vi "HFRR ADV v05 new software.vi"() -> ()   [LabVIEW 2025] (continued)
        n2735 = case shown="True" "OK Button 17" {
          frame False {
          }
          frame True {
            (unwired) 0  # existing file
            w3786 = "Choose a datalog file to open"  # prompt
            n2736 = local write "OK Button 17"(FALSE ("OK Button 17")) -> ()
            n2737 = local read "String"() -> (w3781:string)
            n2738 = String To Path(string=w3781) -> (path=w3782:path)
            n2739 = File Dialog(6:"*.duf" ("pattern"), 7:w3786, 11:w3782) -> (0:w3773:errorcluster, 3:w3792:path)  [unwired: 4 in, 2 out]
            n2740 = Unbundle(w3773) -> ()  [unwired: 3 out]
            n2741 = Open/Create/Replace File "Open File"(file path (use dialog)=w3792) -> (refnum out=w3784:refnum<file>)  [unwired: 5 in, 2 out]
            n2742 = Strip Path(path=w3792) -> (name=w3790:string)  [unwired: 1 out]
            n2743 = Path To String(path=w3792) -> (string=w3775:string)
            n2744 = while {
              tunnel: w3784 -> [w3796]
              i -> [w3793]
              stop <- w3794 continue-if-true
              (unwired) TRUE ("line mode (F)")
              n2745 = Read from Text File "Read File"(file (use dialog)=w3796) -> (text=w3795:string)  [unwired: 3 in, 3 out]
              n2746 = local write "Numeric 16"(w3793) -> ()
              n2747 = String Length(string=w3795) -> (length=w3798:i32)
              n2748 = Greater?(x=w3798, y=1) -> (0:w3794:bool)
            }
            n2749 = local write "String 29"(w3775) -> ()
            n2750 = Search and Replace String(input string=w3775, search string=".duf", replace string=".dgf" ("replace string (\"\")")) -> (result string=→"String Indicator 4":string)  [unwired: 5 in, 3 out]
            n2751 = Match Pattern(string=w3790, regular expression=".dwm") -> (before substring=w3774:string)  [unwired: 1 in, 3 out]
            "String Indicator" <- w3774
            n2752 = Match Pattern(string=w3775, regular expression=".dwm" ("substring (\"\")")) -> (before substring=w3776:string)  [unwired: 1 in, 3 out]
            "String Indicator 3" <- w3776
            n2753 = local write "TITTLE 2"(w3774) -> ()
            n2754 = String To Path(string=w3776) -> (path=w3783:path)
            "path" <- w3783
            n2755 = call <vilib>:"Read Characters From File.vi"("file path (dialog if empty)"=w3783, "start of read offset (chars.:0)"=60 ("start of read offset (chars.: 0)")) -> ("character string"=→"String Indicator 2":string)  [unwired: 4 in, 3 out]
          }
        }
        n2756 = call <vilib>:"Query Available Printers.vi"() -> ("system configured printers"=w3475:string[])  [unwired: 9 in, 2 out]
        "System Configured Printers 2" <- w3475
        n2757 = local read "OK Button 16"() -> (w3472:bool)
        n2758 = case shown="True" "OK Button 16" {
          frame False {
          }
          frame True {
            n2759 = stacked-sequence {
              frame #0 {
                n2760 = local read "Numeric 16"() -> (w3800:i32)
                n2761 = local write "Numeric 10"(w3800) -> ()
              }
              frame #1 {
                n2762 = local read "S.NO"() -> (→"s.NO":string)
                n2763 = local read "String 29"() -> (w3804:string)
                n2764 = String To Path(string=w3804) -> (path=w3803:path)
                n2765 = Open/Create/Replace File "Open File"(file path (use dialog)=w3803) -> (refnum out=w3805:refnum<file>)  [unwired: 5 in, 2 out]
                n2766 = for {
                  N: 16 -> [_]
                  tunnel: w3805 -> [w3812]
                  i -> [w3808]
                  (unwired) TRUE ("line mode (F)")
                  n2767 = Read from Text File "Read File"(file (use dialog)=w3812) -> (text=w3806:string)  [unwired: 3 in, 3 out]
                  n2768 = Match Pattern(string=w3806, regular expression="(") -> (after substring=w3811:string)  [unwired: 1 in, 3 out]
                  n2769 = Match Pattern(string=w3811, regular expression=")") -> (before substring=w3807:string)  [unwired: 1 in, 3 out]
                  n2770 = case shown="1" w3808 {
                    tunnel: w3807 -> [w3813 w3814 _ _ w3815 w3816 w3817 w3819 w3821 w3823 w3825 w3827 w3829 w3831 _]
                    tunnel: w3806 -> [_ _ _ _ _ _ _ _ _ _ _ _ _ _ _]
                    frame 0 {
                      "TITTLE" <- w3813
                    }
                    frame 1 {
                      "Sample ID" <- w3814
                    }
                    frame 2 {
                    }
                    frame 3 {
                    }
                    frame 4 {
                      "Test Date" <- w3815
                    }
                    frame 5 {
                      "Tested by" <- w3816
                    }
                    frame 6 {
                      n2771 = Fract/Exp String To Number(string=w3817) -> (number=→"Humidity before test 2":dbl)  [unwired: 3 in, 1 out]
                    }
                    frame 7 {
                      n2772 = Fract/Exp String To Number(string=w3819) -> (number=→"Temperature before test 2":dbl)  [unwired: 3 in, 1 out]
                    }
                    frame 8 {
                      n2773 = Fract/Exp String To Number(string=w3821) -> (number=→"Humidity after test 2":dbl)  [unwired: 3 in, 1 out]
                    }
                    frame 9 {
                      n2774 = Fract/Exp String To Number(string=w3823) -> (number=→"Temperature after test 2":dbl)  [unwired: 3 in, 1 out]
                    }
                    frame 10 {
                      n2775 = Fract/Exp String To Number(string=w3825) -> (number=→"MWSD 2":dbl)  [unwired: 3 in, 1 out]
                    }
                    frame 11 {
                      n2776 = Fract/Exp String To Number(string=w3827) -> (number=→"AVP 2":dbl)  [unwired: 3 in, 1 out]
                    }
                    frame 12 {
                      n2777 = Fract/Exp String To Number(string=w3829) -> (number=→"HCF 2":dbl)  [unwired: 3 in, 1 out]
                    }
                    frame 13 {
                      n2778 = Fract/Exp String To Number(string=w3831) -> (number=→"WS1.4 2":dbl)  [unwired: 3 in, 1 out]
                    }
                    frame 14, Default {
                    }
                  }
                }
              }
              frame #2 {
              }
            }
            n2779 = local write "OK Button 16"(FALSE ("OK Button 13")) -> ()
          }
        }
        n2780 = Index Array(array=w3475, index="Select Printer 3") -> (element=w3477:string)
        "Selected Printer" <- w3477
        n2781 = case shown="True" w3472 {
          frame False {
          }
          frame True {
            n2782 = flat-sequence {
              frame #0 {
              }
              frame #1 {
                n2783 = Wait (ms)(milliseconds to wait=u32 100) -> ()  [unwired: 1 out]
              }
              frame #2 {
                n2784 = local write "OK Button 16"(FALSE ("Print 3")) -> ()
              }
            }
          }
        }
        n2785 = case shown="True" "Print" {
          tunnel: w3477 -> [_ w3769]
          frame False {
          }
          frame True {
            (unwired) i16 6 ("width (-)")
            (unwired) "TESTED BY : "
            (unwired) "TESTED DATE :"
            (unwired) "SAMPLE ID : "
            (unwired) "SAMPLE DESIGN : "
            w3727 = "\r"
            w3744 = "\r"
            # "add image"
            n2786 = local read "Sample ID"() -> (w3717:string)
            n2787 = local read "Tested by"() -> (w3720:string)
            n2788 = local read "String 34"() -> (w3707:string)
            n2789 = local read "String 45"() -> (w3687:string)
            n2790 = local read "String 35"() -> (w3702:string)
            n2791 = local read "String 37"() -> (w3700:string)
            n2792 = local read "String 32"() -> (w3722:string)
            n2793 = local read "String 36"() -> (w3697:string)
            n2794 = local read "String 31"() -> (w3721:string)
            n2795 = local read "Test Date"() -> (w3718:string)
            n2796 = local read "String 33"() -> (w3723:string)
            n2797 = local read "String 38"() -> (w3693:string)
            n2798 = local read "String 39"() -> (w3690:string)
            n2799 = local write "Print"(FALSE ("Print FF")) -> ()
            n2800 = local read "S 39"() -> (w3705:string)
            n2801 = local read "S 38"() -> (w3712:string)
            n2802 = local read "Temperature before test 2"() -> (w3743:dbl)
            n2803 = local read "Temperature after test 2"() -> (w3733:dbl)
            n2804 = local read "Humidity before test 2"() -> (w3758:dbl)
            n2805 = local read "Humidity after test 2"() -> (w3742:dbl)
            n2806 = local read "MWSD 2"() -> (w3747:dbl)
            n2807 = local read "WS1.4 2"() -> (w3725:dbl)
            n2808 = Concatenate Strings("2)" ("string"), w3707) -> (w3708:string)
            n2809 = Concatenate Strings("3)" ("string"), w3705) -> (w3706:string)
            n2810 = Concatenate Strings("1)" ("string"), w3712) -> (w3711:string)
            n2811 = Concatenate Strings("4)" ("string"), w3702) -> (w3703:string)
            n2812 = Concatenate Strings("5)" ("string"), w3700) -> (w3699:string)
            n2813 = Concatenate Strings("6)" ("string"), w3697) -> (w3696:string)
            n2814 = Concatenate Strings("7)" ("string"), w3693) -> (w3694:string)
            n2815 = Concatenate Strings("8)" ("string"), w3690) -> (w3691:string)
            n2816 = local read "HCF 2"() -> (w3729:dbl)
            n2817 = local read "AVP 2"() -> (w3746:dbl)
            n2818 = local read "s.NO"() -> (w3688:string)
            n2819 = call <vilib>:"New Report.vi"("report type"=enum16{"Standard Report", "HTML"}."Standard Report") -> ("report out"=w3767:refnum<class "NI_report.lvclass">, "error out"=w3766:errorcluster)  [unwired: 13 in]
            n2820 = local read "TITTLE"() -> (w3719:string)
            n2821 = Concatenate Strings(w3744, w3687, w3688, w3744, w3722, w3717, w3744, w3721, w3718, w3744, w3723, w3720, w3744) -> (w3737:string)
            "test by" <- w3737
            n2822 = Number To Fractional String(number=w3743, width (-)=i16 6, precision (6)=i16 2) -> (F-format string=w3732:string)  [unwired: 1 in]
            n2823 = Number To Fractional String(number=w3742, width (-)=i16 6, precision (6)=i16 2) -> (F-format string=w3745:string)  [unwired: 1 in]
            n2824 = Number To Fractional String(number=w3758, width (-)=i16 6, precision (6)=i16 2) -> (F-format string=w3763:string)  [unwired: 1 in]
            n2825 = Number To Fractional String(number=w3747, width (-)=i16 6, precision (6)=i16 2) -> (F-format string=w3749:string)  [unwired: 1 in]
            n2826 = Number To Fractional String(number=w3733, width (-)=i16 6, precision (6)=i16 2) -> (F-format string=w3734:string)  [unwired: 1 in]
            n2827 = Number To Fractional String(number=w3746, width (-)=i16 6, precision (6)=i16 2) -> (F-format string=w3748:string)  [unwired: 1 in]
            n2828 = Number To Fractional String(number=w3729, width (-)=i16 6, precision (6)=i16 2) -> (F-format string=w3728:string)  [unwired: 1 in]
            n2829 = Number To Fractional String(number=w3725, precision (6)=i16 2) -> (F-format string=w3724:string)  [unwired: 2 in]
            n2830 = call-dynamic "Set Report Header Text.vi"("report in"=w3767, "center header text"=w3719, "error in (no error)"=w3766) -> ("report out"=w3738:refnum<class "NI_report.lvclass">, "error out"=w3739:errorcluster)  [unwired: 11 in]
            n2831 = Concatenate Strings(w3727, w3711, w3763, w3727, w3708, w3732, w3727, w3706, w3745, w3727, w3703, w3734, w3727, w3699, w3749, w3727, w3696, w3748, w3727, w3694, w3728, w3727, w3691, w3724) -> (w3715:string)
            "export 2" <- w3715
            n2832 = call-poly <vilib>:"Append Report Text.vi"("report in"=w3738, "text"=w3737, "error in (no error)"=w3739) -> ("report out"=w3741:refnum<class "NI_report.lvclass">, "error out"=w3740:errorcluster)  [unwired: 9 in, 2 out]
            n2833 = local read "test by"() -> (w3714:string)
            n2834 = local read "TITTLE"() -> (w3716:string)
            n2835 = call-poly <vilib>:"Append Report Text.vi"("report in"=w3741, "error in (no error)"=w3740) -> ("report out"=w3762:refnum<class "NI_report.lvclass">, "error out"=w3760:errorcluster)  [unwired: 10 in, 2 out]
            n2836 = Concatenate Strings(w3716, w3715, w3714) -> (→"output":string)
            n2837 = call-poly <vilib>:"Append Report Text.vi"("report in"=w3762, "text"=w3715, "error in (no error)"=w3760) -> ("report out"=w3761:refnum<class "NI_report.lvclass">, "error out"=w3759:errorcluster)  [unwired: 9 in, 2 out]
            n2838 = call-dynamic "Print Report.vi"("report in"=w3761, "printer name (default)"=w3769, "error in (no error)"=w3759) -> ("report out"=w3771:refnum<class "NI_report.lvclass">, "error out"=w3772:errorcluster)  [unwired: 11 in]
            n2839 = call-dynamic "Dispose Report.vi"("report in"=w3771, "error in (no error)"=w3772) -> ()  [unwired: 13 in, 1 out]
          }
        }
        n2840 = case shown="True" "Print 2" {
          frame False {
          }
          frame True {
            n2841 = flat-sequence {
              frame #0 {
                n2842 = local read "s.NO"() -> (→"s.NO 2":string)
                n2843 = Wait (ms)(milliseconds to wait=u32 20) -> ()  [unwired: 1 out]
                n2844 = local read "Sample ID  3"() -> (→"Sample ID  6":string)
                n2845 = local read "Sample ID  4"() -> (→"Sample ID  7":string)
                n2846 = local read "Sample ID"() -> (→"Sample ID  2":string)
                n2847 = local read "Tested by"() -> (→"Tested by 2":string)
                n2848 = local read "Test Date"() -> (→"Test Date 2":string)
                n2849 = local read "Humidity after test 3"() -> (→"Humidity after test 4":dbl)
                n2850 = local read "Ref A Test Date :"() -> (→"TITTLE 4":string)
                n2851 = local read "Temperature before test 3"() -> (w3594:dbl)
                n2852 = local read "Temperature before test 3"() -> (→"Temperature after test 5":dbl)
                n2853 = local read "Temperature after test 3"() -> (→"Temperature after test 4":dbl)
                n2854 = local read "Humidity before test 3"() -> (→"Humidity before test 4":dbl)
                n2855 = local write "Temperature before test 3"(w3594) -> ()
                n2856 = local read "image data"() -> (w3585:T11)
                n2857 = String To Path(string="C:\\LAB-IQ\\im\\Temp_resized.jpg") -> (path=w3586:path)
                "path 2" <- w3586
                n2858 = call <vilib>:"Write JPEG File.vi"("image data"=w3585, "path to JPEG file"=w3586) -> ()  [unwired: 8 in, 2 out]
                "Ref A Test Date :" <- "Ref A Test Date :"
                "Ref B Test Date :" <- "Ref B Test Date :"
                "Ref B Scar Value :" <- "Ref B Scar Value :"
                "Ref A Scar Value :" <- "Ref A Scar Value :"
              }
              frame #1 {
                (unwired) HTML_Report_Image_Alignment."MIDDLE" ("alignment (default)")
                w3622 = u16 0 items=["portrait", "landscape"] ("orientation (portrait)")
                (unwired) HTML_Report_Image_Alignment."ABSMIDDLE" ("alignment (default)")
                (unwired) "TESTED BY : "
                (unwired) "TESTED DATE :"
                (unwired) "SAMPLE ID : "
                (unwired) "SAMPLE DESIGN : "
                w3655 = "\r"
                # "add image"
                n2859 = Wait (ms)(milliseconds to wait=u32 20) -> ()  [unwired: 1 out]
                n2860 = local read "Sample ID  2"() -> (w3648:string)
                n2861 = local read "Wear Scar X"() -> (w3620:dbl)
                "Length ( microns ) 2" <- w3620
                n2862 = local read "Wear Scar Y"() -> (w3619:dbl)
                "Wear Scar Y ( microns ) :" <- w3619
                n2863 = local read "Test Date 2"() -> (w3649:string)
                n2864 = local read "Tested by 2"() -> (w3650:string)
                n2865 = local read "String 46"() -> (w3646:string)
                n2866 = local read "String 48"() -> (w3652:string)
                n2867 = local read "String 47"() -> (w3651:string)
                n2868 = local read "String 49"() -> (w3653:string)
                n2869 = local read "String 10"() -> (w3606:string)
                n2870 = local read "s.NO 2"() -> (w3647:string)
                n2871 = Add(x=w3620, y=w3619) -> (x+y=w3618:dbl)
                n2872 = call <vilib>:"New Report.vi"("report type"=enum16{"Standard Report", "HTML"}."HTML") -> ("report out"=w3626:refnum<class "NI_report.lvclass">, "error out"=w3624:errorcluster)  [unwired: 13 in]
                n2873 = Concatenate Strings(w3655, w3646, w3647, w3655, w3652, w3648, w3655, w3651, w3649, w3655, w3653, w3650, w3655) -> (→"test by 2":string)
                n2874 = Concatenate Strings("C:\\LAB-IQ\\Data\\" ("string"), w3606, ".jpg" ("string")) -> ()  [unwired: 1 out]
                n2875 = Divide(x=w3618, y=2.0) -> (x/y=→"Mean Wear ( microns) :":dbl)
                n2876 = call-dynamic "Set Report Orientation.vi"("report in"=w3626, "orientation (portrait)"=w3622, "error in (no error)"=w3624) -> ("report out"=w3625:refnum<class "NI_report.lvclass">, "error out"=w3623:errorcluster)  [unwired: 11 in]
                n2877 = for {
                  N: 5 -> [_]
                  tunnel: w3625 -> [w3676]
                  tunnel: [w3675] -> w3604
                  tunnel: w3623 -> [w3674]
                  tunnel: [w3673] -> w3603
                  n2878 = call-dynamic "Set Report Tab Width.vi"("report in"=w3676, "error in (no error)"=w3674) -> ("report out"=w3675:refnum<class "NI_report.lvclass">, "error out"=w3673:errorcluster)  [unwired: 12 in]
                }
                n2879 = local read "TITTLE"() -> (w3621:string)
                n2880 = call-dynamic "Set Report Header Text.vi"("report in"=w3604, "center header text"=w3621, "error in (no error)"=w3603) -> ("report out"=w3642:refnum<class "NI_report.lvclass">, "error out"=w3641:errorcluster)  [unwired: 11 in]
                n2881 = for {
                  N: 1 -> [_]
                  tunnel: [w3680] -> w3628
                  tunnel: [w3679] -> w3627
                  tunnel: w3642 -> [w3678]
                  tunnel: w3641 -> [w3677]
                  n2882 = call-dynamic "New Report Line.vi"("report in"=w3678, "error in (no error)"=w3677) -> ("report out"=w3680:refnum<class "NI_report.lvclass">, "error out"=w3679:errorcluster)  [unwired: 12 in]
                }
                n2883 = for {
                  N: 2 -> [_]
                  tunnel: [w3672] -> w3634
                  tunnel: [w3671] -> w3633
                  tunnel: w3628 -> [w3670]
                  tunnel: w3627 -> [w3669]
                  n2884 = call-dynamic "New Report Line.vi"("report in"=w3670, "error in (no error)"=w3669) -> ("report out"=w3672:refnum<class "NI_report.lvclass">, "error out"=w3671:errorcluster)  [unwired: 12 in]
                }
                n2885 = for {
                  N: 25 -> [_]
                  tunnel: w3634 -> [w3668]
                  tunnel: w3633 -> [w3666]
                  tunnel: [w3667] -> w3637
                  tunnel: [w3665] -> w3636
                  n2886 = call-dynamic "Set Report Tab Width.vi"("report in"=w3668, "error in (no error)"=w3666) -> ("report out"=w3667:refnum<class "NI_report.lvclass">, "error out"=w3665:errorcluster)  [unwired: 12 in]
                }
                n2887 = control-ref of="Tab Control 9"() -> (w3632:refnum<vi>)
                n2888 = call-dynamic "Append Control Image to Report.vi"("report in"=w3637, "alignment (default)"=HTML_Report_Image_Alignment."ABSMIDDLE", "ctrl reference"=w3632, "error in (no error)"=w3636) -> ("report out"=w3631:refnum<class "NI_report.lvclass">, "error out"=w3630:errorcluster)  [unwired: 8 in, 2 out]
                n2889 = for {
                  N: 3 -> [_]
                  tunnel: [w3664] -> w3615
                  tunnel: [w3663] -> w3614
                  tunnel: w3631 -> [w3662]
                  tunnel: w3630 -> [w3661]
                  n2890 = call-dynamic "New Report Line.vi"("report in"=w3662, "error in (no error)"=w3661) -> ("report out"=w3664:refnum<class "NI_report.lvclass">, "error out"=w3663:errorcluster)  [unwired: 12 in]
                }
                n2891 = for {
                  N: 100 -> [_]
                  tunnel: w3615 -> [w3660]
                  tunnel: w3614 -> [w3658]
                  tunnel: [w3659] -> w3611
                  tunnel: [w3657] -> w3609
                  n2892 = call-dynamic "Set Report Tab Width.vi"("report in"=w3660, "error in (no error)"=w3658) -> ("report out"=w3659:refnum<class "NI_report.lvclass">, "error out"=w3657:errorcluster)  [unwired: 12 in]
                }
                n2893 = String To Path(string="C:\\LAB-IQ\\im\\Temp_resized.jpg") -> (path=w3601:path)
                n2894 = call-poly <vilib>:"Append Image to Report.vi"("report in"=w3611, "path or URL of image"=w3601, "error in (no error)"=w3609) -> ("report out"=w3610:refnum<class "NI_report.lvclass">, "error out"=w3608:errorcluster)  [unwired: 9 in, 2 out]
                n2895 = call-poly <vilib>:"Open HTML Report in Browser.vi"("report in"=w3610, "error in (no error)"=w3608) -> ("report out"=w3645:refnum<class "NI_report.lvclass">, "error out"=w3644:errorcluster)  [unwired: 11 in, 1 out]
                n2896 = call-dynamic "Dispose Report.vi"("report in"=w3645, "error in (no error)"=w3644) -> ()  [unwired: 13 in, 1 out]
              }
              frame #2 {
              }
              frame #3 {
                n2897 = disable-structure shown="Disabled" {
                  frame Disabled {
                    n2898 = local read "String 10"() -> (w3685:string)
                    n2899 = Concatenate Strings("C:\\LAB-IQ-NXT\\Data\\" ("string"), w3685, ".jpg" ("string")) -> (w3683:string)
                    n2900 = String To Path(string=w3683) -> (path=w3682:path)
                    n2901 = Delete(path (use dialog)=w3682) -> ()  [unwired: 4 in, 3 out]
                  }
                  frame Enabled {
                  }
                }
                n2902 = local write "Print 2"(FALSE ("Print")) -> ()
              }
            }
          }
        }
      }
    }
    n2903 = property on="SetTemp" class="DigNum (strict)"("Disabled"=w1631) -> ()  [unwired: 2 in, 2 out]
    n2904 = Multiply(x=w1621, y=w1623) -> (x*y=w1622:dbl)
    n2905 = local read "MWSD"() -> (w1620:dbl)
    n2906 = Add(x=w1622, y=w1620) -> (x+y=→"WS1.4":dbl)
    n2907 = Wait (ms)(milliseconds to wait=u32 50) -> ()  [unwired: 1 out]
    n2908 = Wait (ms)(milliseconds to wait=u32 50) -> ()  [unwired: 1 out]
    n2909 = local read "Quit"() -> (w1619:bool)
  }
  n2910 = VISA Close(VISA resource name=w52, error in (no error)=w51) -> (error out=w49:errorcluster)
  n2911 = call <vilib>:"Clear Errors.vi"("error in (no error)"=w49) -> ()  [unwired: 5 in, 2 out]
  n2912 = VISA Close(VISA resource name=w37, error in (no error)=w36) -> ()  [unwired: 1 out]
  n2913 = while {
    tunnel: [w3844] -> w46
    shift-right: [w3837] -> _
    shift-left: 0.0 -> [w3840]
    shift-right: [w3836] -> _
    shift-left: 0.0 -> [w3839]
    shift-right: [w3835] -> _
    shift-left: 400.0 ("vc_cmd") -> [w3838]
    stop <- w3844 stop-if-true
    # "PID LOGIC"
    n2914 = local read "RUN"() -> (w3842:bool)
    n2915 = local read "Auto Start Test"() -> (w3841:bool)
    n2916 = local read "START TEMP"() -> (w3833:bool)
    n2917 = Or(x=w3842, y=w3841) -> (x .or. y?=w3843:bool)
    n2918 = And(x=w3843, y=w3833) -> (x .and. y?=w3834:bool)
    n2919 = Wait (ms)(milliseconds to wait=u32 20) -> ()  [unwired: 1 out]
    n2920 = case shown="True" w3834 {
      tunnel: [400.0 ("out_vc_cmd") w3864] -> w3835
      tunnel: [w3847 w3866] -> w3836
      tunnel: [w3847 w3865] -> w3837
      tunnel: w3840 -> [_ w3855]
      tunnel: w3839 -> [_ w3854]
      tunnel: w3838 -> [_ w3853]
      frame False {
        w3847 = 0.0 ("error_out")
      }
      frame True {
        n2921 = local read "Set Strk"() -> (w3850:dbl)
        n2922 = local read "LVDT STROKE"() -> (w3848:dbl)
        n2923 = Add(x=w3850, y="Add up Stroke") -> (x+y=w3851:dbl)
        n2924 = formula code="// Zero-Hardcode Explicit Positional-Form PID Engine\n// Inputs: target_stroke, measured_stroke, dt, prev_error, integral_accumulator_in, prev_vc_cmd\n//         kp, ki, kd, max_step_change, max_amplitude, min_amplitude, startup_cmd\n// Outputs: vc_cmd, error_out, out_error, integral_accumulator_out, out_vc_cmd\n\n// 1. Calculate Tracking Error\nfloat current_error = target_stroke - measured_stroke;\nerror_out = current_error;\n\n// 2. Compute Proportional Term\nfloat p_term = kp * current_error;\n\n// 3. Compute Derivative Term\nfloat d_term = 0.0;\nif (dt > 0.0) {\n    d_term = kd * ((current_error - prev_error) / dt);\n}\n\n// 4. Update and Accumulate Integral Term\nfloat current_integral = integral_accumulator_in + (current_error * dt);\nfloat i_term = ki * current_integral;\n\n// 5. Calculate Ideal Target Command\nfloat ideal_command = startup_cmd + p_term + i_term + d_term;\n\n// 6. Anti-Windup Protection (Back-calculation method)\nif (ideal_command > max_amplitude) {\n    float excess = ideal_command - max_amplitude;\n    if (ki > 0.0) {\n        current_integral -= excess / ki;\n    }\n    ideal_command = max_amplitude;\n} else if (ideal_command < min_amplitude) {\n    float excess = ideal_command - min_amplitude;\n    if (ki > 0.0) {\n        current_integral -= excess / ki;\n    }\n    ideal_command = min_amplitude;\n}\n\n// 7. Apply Loop Rate Limiting (Protects voice coil from large voltage steps)\nfloat raw_adjustment = ideal_command - prev_vc_cmd;\n\nif (raw_adjustment > max_step_change) {\n    raw_adjustment = max_step_change;\n} else if (raw_adjustment < -max_step_change) {\n    raw_adjustment = -max_step_change;\n}\n\nfloat next_vc_cmd = prev_vc_cmd + raw_adjustment;\n\n// Final Output Safety Safeguard Clamping\nif (next_vc_cmd > max_amplitude) {\n    next_vc_cmd = max_amplitude;\n} else if (next_vc_cmd < min_amplitude) {\n    next_vc_cmd = min_amplitude;\n}\n\n// 8. Map to Shift Registers for memory persistence\nvc_cmd = next_vc_cmd;\nout_error = current_error;                     \nintegral_accumulator_out = current_integral;  \nout_vc_cmd = next_vc_cmd;"("target_stroke"=w3851, "measured_stroke"=w3848, "dt"="dt", "integral_accumulator_in"=w3854, "prev_error"=w3855, "prev_vc_cmd"=w3853, "kp"="kp", "ki"="ki", "kd"="kd", "max_step_change"="max_step_change", "max_amplitude"="max_amplitude", "min_amplitude"="min_amplitude", "startup_cmd"="startup_cmd") -> ("vc_cmd"=w3870:dbl, "out_error"=w3865:dbl, "integral_accumulator_out"=w3866:dbl, "out_vc_cmd"=w3864:dbl)  [unwired: 1 out]
        "output Vpp" <- w3870
        n2925 = Number To Fractional String(number=w3870, precision (6)=i16 1) -> (F-format string=w3868:string)  [unwired: 2 in]
        n2926 = Concatenate Strings("DAC;" ("string"), w3868) -> (w3852:string)
        n2927 = local write "Command"(w3852) -> ()
        "prev_error" <- w3855
        "integral_accumulator_in" <- w3854
        "prev_vc_cmd" <- w3853
      }
    }
    n2928 = local read "Quit"() -> (w3844:bool)
  }
  n2929 = Or(x=w42, y=w41) -> (x .or. y?=w43:bool)
  n2930 = Or(x=w39, y=w43) -> (x .or. y?=w48:bool)
  n2931 = control-ref of="new picture"() -> ()  [unwired: 1 out]
  n2932 = Or(x=w54, y=w48) -> (x .or. y?=w45:bool)
  n2933 = Or(x=w45, y=w46) -> (x .or. y?=w40:bool)
  n2934 = while {
    tunnel: [w3871] -> w53
    i -> [w3878]
    stop <- w3871 stop-if-true
    n2935 = local read "Quit"() -> (w3871:bool)
    n2936 = Equal To 0?(x=w3878) -> (x = 0?=w3876:bool)
    n2937 = call "Elapsed Time3"("Time Target (s)"=45.0, "Auto Reset"=TRUE) -> ("Time has Elapsed"=w3875:bool)  [unwired: 10 in, 7 out]
    n2938 = Wait (ms)(milliseconds to wait=u32 50) -> ()  [unwired: 1 out]
    n2939 = Or(x=w3875, y=w3876) -> (x .or. y?=w3877:bool)
    n2940 = case shown="True" w3877 {
      frame False {
      }
      frame True {
        n2941 = call <vilib>:"System Exec.vi"("run minimized? (F)"=TRUE, "error in (no error)"="error in (no error)", "command line"="powercfg.exe -change -monitor-timeout-ac 0") -> ("error out"=w3889:errorcluster)  [unwired: 5 in, 3 out]
        n2942 = call <vilib>:"System Exec.vi"("run minimized? (F)"=TRUE, "error in (no error)"=w3889, "command line"="powercfg.exe -change -disk-timeout-ac 0") -> ("error out"=w3888:errorcluster)  [unwired: 5 in, 3 out]
        n2943 = call <vilib>:"System Exec.vi"("run minimized? (F)"=TRUE, "error in (no error)"=w3888, "command line"="powercfg.exe -change -standby-timeout-ac 0") -> ("error out"=w3887:errorcluster)  [unwired: 5 in, 3 out]
        n2944 = call <vilib>:"System Exec.vi"("run minimized? (F)"=TRUE, "error in (no error)"=w3887, "command line"="powercfg.exe -change -hibernate-timeout-ac 0") -> ("error out"=w3886:errorcluster)  [unwired: 5 in, 3 out]
        n2945 = call <vilib>:"Simple Error Handler.vi"("error in (no error)"=w3886) -> ("error out"=w3892:errorcluster)  [unwired: 4 in, 4 out]
        n2946 = call <vilib>:"Clear Errors.vi"("error in (no error)"=w3892) -> ("error out"=→"error out":errorcluster)  [unwired: 5 in, 1 out]
      }
    }
  }
  n2947 = Compound Arithmetic op=OR(w56, w40, w53) -> (w55:bool)
  n2948 = flat-sequence {
    tunnel: w55 -> [_]
    tunnel: [w3894] -> w17
    tunnel: w17 -> [_]
    frame #0 {
      n2949 = call "CLOSE CONNECTION.vi"() -> ("error out"=w3894:errorcluster)  [unwired: 11 in]
    }
    frame #1 {
      n2950 = Quit LabVIEW(quit? (T)=TRUE) -> ()
      n2951 = local write "Quit"(FALSE ("EXIT")) -> ()
    }
  }
  n2952 = property on="Heater Button" class="Bool (strict)"("Visible"=TRUE) -> ()  [unwired: 2 in, 2 out]
  n2953 = disable-structure shown="Disabled" {
    disable-tunnel: _ -> [w3900 _]
    disable-tunnel: _ -> [w3897 _]
    disable-tunnel: _ -> [w3898 _]
    frame Disabled {
      n2954 = disable-structure shown="Disabled" {
        disable-tunnel: [w3907 _] -> w3899
        frame Disabled {
          n2955 = while {
            shift-right: [w3949] -> w3905
            shift-left: errorcluster {"status"=TRUE, "code"=0, "source"="Init"} ("error out") -> [w3914]
            shift-right: [w3948] -> w3904
            shift-left: _ -> [w3915]
            shift-right: [w3947] -> _
            shift-left: "" -> [w3946]
            tunnel: [w3908] -> w3907
            shift-right: ["Set Rh"] -> _
            shift-left: 0.0 ("Set Rh") -> [w3940]
            tunnel: [w3917] -> _
            i -> [w3917]
            stop <- w3908 stop-if-true
            n2956 = flat-sequence {
              tunnel: w3914 -> [w3952]
              tunnel: [w3952] -> w3913
              frame #0 {
                n2957 = Wait (ms)(milliseconds to wait=u32 200) -> ()  [unwired: 1 out]
              }
            }
            n2958 = local read "Com Port 3"() -> (w3916:refnum<visa-resource-name>)
            n2959 = local read "Humidity Str Rec"() -> (w3918:string)
            n2960 = Not Equal?(x="Set Rh", y=w3940) -> (x != y?=w3945:bool)
            n2961 = Number To Decimal String(number="Set Rh") -> (decimal integer string=w3943:string)  [unwired: 1 in]
            n2962 = Not Equal?(x=w3916, y=w3915) -> (x != y?=w3911:bool)
            n2963 = Concatenate Strings("#setPoint00" ("string"), w3943) -> (w3944:string)
            n2964 = case shown="False" w3945 {
              tunnel: w3944 -> [_ w3964]
              frame False {
                n2965 = local read "Humidity"() -> (w3961:bool)
                n2966 = case shown="True" w3961 {
                  frame False {
                    n2967 = local write "Humidity Str Send"("stop" ("Humidity Str Send")) -> ()
                  }
                  frame True {
                    n2968 = local write "Humidity Str Send"("start" ("Humidity Str Send")) -> ()
                  }
                }
              }
              frame True {
                n2969 = local write "Humidity Str Send"(w3964) -> ()
              }
            }
            n2970 = Or(x=w3911) -> (y=w3909:bool, x .or. y?=w3910:bool)
            n2971 = String Subset(string=w3918, offset (0)=7) -> (substring=w3933:string)  [unwired: 1 in]
            n2972 = Match Pattern(string=w3918, regular expression="?") -> (offset past match=w3936:i32)  [unwired: 1 in, 3 out]
            n2973 = Match Pattern(string=w3918, regular expression="v") -> (offset past match=w3939:i32)  [unwired: 1 in, 3 out]
            n2974 = case shown="True" w3910 {
              tunnel: w3913 -> [w3950 _]
              tunnel: [w3950 errorcluster {"status"=TRUE, "code"=0, "source"="Init"} ("error out")] -> w3912
              frame False {
              }
              frame True {
              }
            }
            n2975 = Equal?(x=w3936, y=-1) -> (x = y?=w3920:bool)
            n2976 = Match Pattern(string=w3933, regular expression="g") -> (after substring=w3934:string, offset past match=w3925:i32)  [unwired: 1 in, 2 out]
            n2977 = Match Pattern(string=w3933, regular expression="y") -> (after substring=w3932:string, offset past match=w3926:i32)  [unwired: 1 in, 2 out]
            n2978 = Greater?(x=w3926, y=w3925) -> (0:w3931:bool)
            n2979 = Greater Or Equal To 0?(x=w3926) -> (x >= 0?=w3923:bool)
            n2980 = Greater Or Equal To 0?(x=w3925) -> (x >= 0?=w3924:bool)
            n2981 = Or(x=w3923, y=w3924) -> (x .or. y?=w3922:bool)
            n2982 = Greater Or Equal To 0?(x=w3939) -> (x >= 0?=w3921:bool)
            n2983 = Select(t=w3932, s=w3931, f=w3934) -> (s? t:f=w3927:string)
            n2984 = case shown="Error" w3912 {
              selector: w3912 -> [w3977 w4023]
              tunnel: [w3975 w4016] -> w3949
              tunnel: w3915 -> [w3978 w4022]
              tunnel: [w3976 w4025] -> w3948
              tunnel: w3946 -> [w3965 w4024]
              tunnel: [w3972 w4024] -> w3947
              frame No Error {
                n2985 = call "Elapsed Time7"() -> ("Time has Elapsed"=w3971:bool)  [unwired: 12 in, 7 out]
                n2986 = Not Equal?(x="Humidity Str Send", y=w3965) -> (x != y?=w3967:bool)
                n2987 = Or(x=w3967, y=w3971) -> (x .or. y?=w3970:bool)
                n2988 = Select(t="Humidity Str Send", s=w3967, f="vals" ("regular expression")) -> (s? t:f=w3966:string)
                n2989 = Or(x=w3970, y="Send") -> (x .or. y?=w3974:bool)
                n2990 = case shown="True" w3974 {
                  tunnel: [w3981 w3986] -> w3975
                  tunnel: w3978 -> [w3980 w3994]
                  tunnel: w3977 -> [w3981 w3993]
                  tunnel: [w3980 w3987] -> w3976
                  tunnel: w3966 -> [_ w3992]
                  tunnel: [w3979 w3983] -> w3972
                  tunnel: "Humidity Str Send" -> [_ w3984]
                  tunnel: w3967 -> [_ w3985]
                  tunnel: w3965 -> [w3979 w3982]
                  frame False {
                  }
                  frame True {
                    n2991 = flat-sequence {
                      tunnel: w3994 -> [w4002]
                      tunnel: w3993 -> [w4001]
                      tunnel: w3992 -> [w3998]
                      tunnel: [w4000] -> w3991
                      tunnel: [w3999] -> w3990
                      tunnel: w3991 -> [w4005]
                      tunnel: w3990 -> [w4004]
                      tunnel: [w4005] -> w3989
                      tunnel: [w4004] -> w3988
                      tunnel: w3989 -> [w4012]
                      tunnel: w3988 -> [w4011]
                      tunnel: [w4010] -> w3987
                      tunnel: [w4009] -> w3986
                      frame #0 {
                        n2992 = local write "Ser Led"(TRUE ("Boolean 4")) -> ()
                        n2993 = Concatenate Strings(w3998, "\r") -> (w3997:string)
                        n2994 = VISA Write(VISA resource name=w4002, write buffer=w3997, error in (no error)=w4001) -> (VISA resource name out=w4000:refnum<visa-resource-name>, error out=w3999:errorcluster)  [unwired: 1 out]
                      }
                      frame #1 {
                        n2995 = Wait (ms)(milliseconds to wait="wait") -> ()  [unwired: 1 out]
                      }
                      frame #2 {
                        w4007 = FALSE ("Send")
                        n2996 = property class="Instr"(reference=w4012, error in=w4011) -> (reference out=w4013:refnum<visa-resource-name>, error out=w4014:errorcluster, "Serial Settings:Number of Bytes at Serial Port"=w4006:u32)
                        n2997 = local write "Send"(w4007) -> ()
                        n2998 = local write "Ser Led"(w4007) -> ()
                        n2999 = VISA Read(VISA resource name=w4013, byte count=w4006, error in (no error)=w4014) -> (VISA resource name out=w4010:refnum<visa-resource-name>, read buffer=→"Humidity Str Rec":string, error out=w4009:errorcluster)  [unwired: 1 out]
                      }
                    }
                    n3000 = Select(t=w3984, s=w3985, f=w3982) -> (s? t:f=w3983:string)
                  }
                }
              }
              frame Error {
                w4030 = u16 0 items=["None"=0, "XON/XOFF"=1, "RTS/CTS"=2, "DTR/DSR"=4] ("flow control")
                w4026 = u16 0 items=["None", "Odd", "Even", "Mark", "Space"] ("parity")
                w4029 = u16 10 items=["1.0"=10, "1.5"=15, "2.0"=20] ("stop bits")
                n3001 = VISA Close(VISA resource name=w4022, error in (no error)=w4023) -> (error out=w4021:errorcluster)
                n3002 = local write "humid"("" ("humid")) -> ()
                n3003 = local write "Humidity Str Rec"("" ("Humidity Str Rec")) -> ()
                n3004 = call <vilib>:"Clear Errors.vi"("error in (no error)"=w4021) -> ("error out"=w4020:errorcluster)  [unwired: 5 in, 1 out]
                n3005 = local read "Com Port 3"() -> (w4019:refnum<visa-resource-name>)
                n3006 = call-poly "VISA Configure Serial Port"("VISA resource name"=w4019, "timeout (10sec)"=u32 1000, "termination char\n(0xA = '\\n' = LF)"=u8 10 ("termination char\n(0xA = '\\n' = LF)"), "Enable Termination\nChar (T)"=FALSE ("Enable Termination Char (T)"), "data bits (8)"=u16 8 ("data bits"), "parity (0:none)"=w4026, "error in (no error)"=w4020, "stop bits (10: 1 bit)"=w4029, "flow control (0:none)"=w4030) -> ("VISA resource name out"=w4025:refnum<visa-resource-name>, "baud rate (9600)"=w4017:u32, "error out"=w4016:errorcluster)  [unwired: 4 in]
              }
            }
            n3007 = Compound Arithmetic op=AND(w3921, w3920, w3922) -> (w3919:bool)
            n3008 = case shown="True" w3919 {
              tunnel: w3918 -> [_ _]
              tunnel: w3927 -> [_ w3957]
              frame False {
              }
              frame True {
                w3955 = " " ("regular expression")
                n3009 = Match Pattern(string=w3957, regular expression=" ") -> (after substring=w3959:string)  [unwired: 1 in, 3 out]
                n3010 = Match Pattern(string=w3959, regular expression=w3955) -> (before substring=→"humid":string, after substring=w3956:string)  [unwired: 1 in, 2 out]
                n3011 = Match Pattern(string=w3956, regular expression=w3955) -> (before substring=→"temp_@Rh sensor":string)  [unwired: 1 in, 3 out]
              }
            }
            n3012 = local read "Quit"() -> (w3908:bool)
          }
          n3013 = VISA Close(VISA resource name=w3904, error in (no error)=w3905) -> (error out=w3901:errorcluster)
          n3014 = call <vilib>:"Clear Errors.vi"("error in (no error)"=w3901) -> ()  [unwired: 5 in, 2 out]
        }
        frame Enabled {
        }
      }
    }
    frame Enabled {
    }
  }
  n3015 = while {
    tunnel: [w4037] -> _
    i -> [w4037]
    stop <- w4033 stop-if-true
    # "Langauage selection"
    n3016 = Equal?(x="Lan flag", y=22.0) -> ()  [unwired: 1 out]
    n3017 = disable-structure shown="Disabled" {
      frame Disabled {
        n3018 = stacked-sequence {
          frame #0 {
            n3019 = case shown="\"Russian\"" "Language Selection" {
              tunnel: [0 1] -> w4039
              frame "English", Default {
              }
              frame "Russian" {
              }
            }
            n3020 = for {
              N: 130 -> [_]
              tunnel: "Table" -> [w4048]
              tunnel: w4039 -> [w4047]
              i -> [w4046]
              n3021 = Index Array(array=w4048, index (row)=w4046, index (col)=w4047) -> (element=w4045:string)
              n3022 = case shown="123" w4046 {
                tunnel: w4045 -> [w4049 w4050 _ w4051 w4052 w4053 w4054 w4055 w4056 w4057 w4058 w4059 w4060 w4061 w4062 w4063 w4064 w4065 w4066 w4067 w4068 w4069 w4070 w4071 w4072 w4073 w4074 w4075 w4076 _ _ w4077 w4078 w4079 w4080 w4081 w4082 w4091 w4098 w4105 w4112 w4116 w4119 w4122 w4124 w4126 w4127 w4128 w4129 w4130 w4131 w4132 w4133 w4134 w4135 w4136 w4137 w4138 w4139 w4140 w4141 w4142 w4143 w4144 w4145 w4146 w4147 w4148 w4149 w4150 w4151 w4152 w4153 w4154 w4155 w4156 w4157 w4158 w4159 w4160 w4161 w4162 w4163 w4164 w4165 w4166 w4167 w4168 w4169 w4170 w4171 w4172 w4173 w4174 w4175 w4176 w4177 w4178 w4179 w4180 w4181 w4182 w4183 w4184 w4185 _ w4186 w4187 w4188 w4189 w4190 w4191 w4192 w4193 w4194 w4195 w4196 w4197 w4198 _ w4199 w4200 w4201 w4202 w4203 w4204 _]
                frame 0 {
                  n3023 = local write "S"(w4049) -> ()
                }
                frame 1 {
                  n3024 = local write "S 2"(w4050) -> ()
                }
                frame 2 {
                }
                frame 3 {
                  n3025 = local write "S 4"(w4051) -> ()
                }
                frame 4 {
                  n3026 = property on="FILE" class="Str"("Caption.Text"=w4052) -> ()  [unwired: 2 in, 2 out]
                }
                frame 5 {
                  n3027 = property on="Fuel Discription :" class="Str"("Caption.Text"=w4053) -> ()  [unwired: 2 in, 2 out]
                }
                frame 6 {
                  n3028 = property on="Remarks :" class="Str"("Caption.Text"=w4054) -> ()  [unwired: 2 in, 2 out]
                }
                frame 7 {
                  n3029 = property on="Save & Continue" class="Bool (strict)"("Boolean Text.Text"=w4055) -> ()  [unwired: 2 in, 2 out]
                }
                frame 8 {
                }
                frame 9 {
                  n3030 = property on="Set Hz" class="DigNum (strict)"("Caption.Text"=w4057) -> ()  [unwired: 2 in, 2 out]
                }
                frame 10 {
                  "String 3" <- w4058
                }
                frame 11 {
                  n3031 = property on="NORMAL LOAD" class="DigNum (strict)"("Caption.Text"=w4059) -> ()  [unwired: 2 in, 2 out]
                }
                frame 12 {
                  "String 5" <- w4060
                }
                frame 13 {
                  n3032 = property on="Set Temp" class="DigNum (strict)"("Caption.Text"=w4061) -> ()  [unwired: 2 in, 2 out]
                }
                frame 14 {
                  n3033 = local write "S 15"(w4062) -> ()
                }
                frame 15 {
                  n3034 = property on="Set Rh" class="DigNum (strict)"("Caption.Text"=w4063) -> ()  [unwired: 2 in, 2 out]
                }
                frame 16 {
                  "String 13" <- w4064
                  "String 26" <- w4064
                }
                frame 17 {
                  n3035 = local write "S 18"(w4065) -> ()
                }
                frame 18 {
                  "String 17" <- w4066
                }
                frame 19 {
                  n3036 = property on="test time" class="DigNum (strict)"("Caption.Text"=w4067) -> ()  [unwired: 2 in, 2 out]
                }
                frame 20 {
                  "String 18" <- w4068
                  "String 22" <- w4068
                }
                frame 21 {
                  n3037 = property on="Elapsed time" class="DigNum (strict)"("Caption.Text"=w4069) -> ()  [unwired: 2 in, 2 out]
                }
                frame 22 {
                  n3038 = property on="Samplingtime 2" class="DigNum (strict)"("Caption.Text"=w4070) -> ()  [unwired: 2 in, 2 out]
                }
                frame 23 {
                  "String 21" <- w4071
                }
                frame 24 {
                  n3039 = property on="Countdown" class="DigNum (strict)"("Caption.Text"=w4072) -> ()  [unwired: 2 in, 2 out]
                }
                frame 25 {
                  n3040 = property on="Countdown 2" class="DigNum (strict)"("Caption.Text"=w4073) -> ()  [unwired: 2 in, 2 out]
                }
                frame 26 {
                  n3041 = property on="Engage" class="Bool (strict)"("Boolean Text.Text"=w4074) -> ()  [unwired: 2 in, 2 out]
                }
                frame 27 {
                  n3042 = property on="Boolean  4" class="Bool (strict)"("Boolean Text.Text"=w4075) -> ()  [unwired: 2 in, 2 out]
                }
                frame 28 {
                  n3043 = property on="Test \nStatus" class="Bool (strict)"("Boolean Text.Text"=w4076) -> ()  [unwired: 2 in, 2 out]
                }
                frame 29 {
                }
                frame 30 {
                }
                frame 31 {
                }
                frame 32 {
                  n3044 = property on="RSTCOF" class="Bool"("Boolean Text.Text"=w4078) -> ()  [unwired: 2 in, 2 out]
                  n3045 = property on="RST FF" class="Bool"("Boolean Text.Text"=w4078) -> ()  [unwired: 2 in, 2 out]
                  n3046 = property on="RST TEMP" class="Bool"("Boolean Text.Text"=w4078) -> ()  [unwired: 2 in, 2 out]
                  n3047 = property on="RSTV1 3" class="Bool"("Boolean Text.Text"=w4078) -> ()  [unwired: 2 in, 2 out]
                  n3048 = property on="rstv2" class="Bool"("Boolean Text.Text"=w4078) -> ()  [unwired: 2 in, 2 out]
                  n3049 = property on="RSTV1 2" class="Bool"("Boolean Text.Text"=w4078) -> ()  [unwired: 2 in, 2 out]
                  n3050 = property on="RST CP" class="Bool"("Boolean Text.Text"=w4078) -> ()  [unwired: 2 in, 2 out]
                }
                frame 33 {
                  "S 61" <- w4079
                }
                frame 34 {
                  "String 23" <- w4080
                }
                frame 35 {
                  n3051 = property on="Rh Before" class="DigNum (strict)"("Caption.Text"=w4081) -> ()  [unwired: 2 in, 2 out]
                }
                frame 36 {
                  n3052 = Match Pattern(string=w4082, regular expression=",") -> (before substring=→"bs":string, after substring=→"as":string)  [unwired: 1 in, 2 out]
                  n3053 = property on="Rh After" class="DigNum (strict)"("Caption.Text"=w4082) -> ()  [unwired: 2 in, 2 out]
                }
                frame 37 {
                  n3054 = Match Pattern(string=w4091, regular expression=",") -> (before substring=w4090:string, after substring=w4089:string)  [unwired: 1 in, 2 out]
                  "bs" <- w4090
                  "as" <- w4089
                  n3055 = Concatenate Strings(w4090, w4089) -> (w4086:string)
                  n3056 = property on="Humidity before test 2" class="DigNum (strict)"("Caption.Text"=w4086) -> ()  [unwired: 2 in, 2 out]
                  n3057 = property on="Humidity before test" class="DigNum (strict)"("Caption.Text"=w4086) -> ()  [unwired: 2 in, 2 out]
                  n3058 = Concatenate Strings(w4086, "=" ("string")) -> (w4087:string)
                  n3059 = local write "S 38"(w4087) -> ()
                }
                frame 38 {
                  n3060 = Match Pattern(string=w4098, regular expression=",") -> (before substring=w4097:string, after substring=w4096:string)  [unwired: 1 in, 2 out]
                  "bs" <- w4097
                  "as" <- w4096
                  n3061 = Concatenate Strings(w4097, w4096) -> (w4093:string)
                  n3062 = property on="Humidity after test 2" class="DigNum (strict)"("Caption.Text"=w4093) -> ()  [unwired: 2 in, 2 out]
                  n3063 = Concatenate Strings(w4093, "=" ("string")) -> (w4095:string)
                  n3064 = property on="Humidity after test" class="DigNum (strict)"("Caption.Text"=w4093) -> ()  [unwired: 2 in, 2 out]
                  n3065 = local write "S 39"(w4095) -> ()
                }
                frame 39 {
                  n3066 = Match Pattern(string=w4105, regular expression=",") -> (before substring=w4104:string, after substring=w4103:string)  [unwired: 1 in, 2 out]
                  "bs" <- w4104
                  "as" <- w4103
                  n3067 = Concatenate Strings(w4104, w4103) -> (w4100:string)
                  n3068 = property on="Temperature before test 2" class="DigNum (strict)"("Caption.Text"=w4100) -> ()  [unwired: 2 in, 2 out]
                  n3069 = property on="Temperature before test" class="DigNum (strict)"("Caption.Text"=w4100) -> ()  [unwired: 2 in, 2 out]
                  n3070 = Concatenate Strings(w4100, "=" ("string")) -> (→"String 34":string)
                }
                frame 40 {
                  n3071 = Match Pattern(string=w4112, regular expression=",") -> (before substring=w4111:string, after substring=w4110:string)  [unwired: 1 in, 2 out]
                  "bs" <- w4111
                  "as" <- w4110
                  n3072 = Concatenate Strings(w4111, w4110) -> (w4107:string)
                  n3073 = property on="Temperature after test 2" class="DigNum (strict)"("Caption.Text"=w4107) -> ()  [unwired: 2 in, 2 out]
                  n3074 = Concatenate Strings(w4107, "=" ("string")) -> (→"String 35":string)
                  n3075 = property on="Temperature after test" class="DigNum (strict)"("Caption.Text"=w4107) -> ()  [unwired: 2 in, 2 out]
                }
                frame 41 {
                  n3076 = property on="AVP" class="DigNum (strict)"("Caption.Text"=w4116) -> ()  [unwired: 2 in, 2 out]
                  n3077 = property on="AVP 2" class="DigNum (strict)"("Caption.Text"=w4116) -> ()  [unwired: 2 in, 2 out]
                  n3078 = Concatenate Strings(w4116, "=" ("string")) -> (→"String 36":string)
                }
                frame 42 {
                  n3079 = property on="MWSD" class="DigNum (strict)"("Caption.Text"=w4119) -> ()  [unwired: 2 in, 2 out]
                  n3080 = property on="MWSD 2" class="DigNum (strict)"("Caption.Text"=w4119) -> ()  [unwired: 2 in, 2 out]
                  n3081 = Concatenate Strings(w4119, "=" ("string")) -> (→"String 37":string)
                }
                frame 43 {
                  n3082 = property on="HCF 2" class="DigNum (strict)"("Caption.Text"=w4122) -> ()  [unwired: 2 in, 2 out]
                  n3083 = property on="HCF" class="DigNum (strict)"("Caption.Text"=w4122) -> ()  [unwired: 2 in, 2 out]
                  n3084 = Concatenate Strings(w4122, "=" ("string")) -> (→"String 38":string)
                }
                frame 44 {
                  n3085 = Concatenate Strings(w4124, "=" ("string")) -> (→"String 39":string)
                  n3086 = property on="WS1.4 2" class="DigNum (strict)"("Caption.Text"=w4124) -> ()  [unwired: 2 in, 2 out]
                  n3087 = property on="WS1.4" class="DigNum (strict)"("Caption.Text"=w4124) -> ()  [unwired: 2 in, 2 out]
                }
                frame 45 {
                  n3088 = property on="Save Results" class="Bool (strict)"("Boolean Text.Text"=w4126) -> ()  [unwired: 2 in, 2 out]
                }
                frame 46 {
                  n3089 = local write "S 47"(w4127) -> ()
                }
                frame 47 {
                  n3090 = local write "S 48"(w4128) -> ()
                }
                frame 48 {
                  n3091 = local write "S 49"(w4129) -> ()
                }
                frame 49 {
                  n3092 = local write "S 50"(w4130) -> ()
                }
                frame 50 {
                  n3093 = local write "S 51"(w4131) -> ()
                }
                frame 51 {
                  n3094 = local write "S 52"(w4132) -> ()
                }
                frame 52 {
                  n3095 = local write "S 53"(w4133) -> ()
                }
                frame 53 {
                  n3096 = local write "S 54"(w4134) -> ()
                }
                frame 54 {
                  n3097 = local write "S 55"(w4135) -> ()
                }
                frame 55 {
                  n3098 = local write "S 56"(w4136) -> ()
                }
                frame 56 {
                  n3099 = local write "S 57"(w4137) -> ()
                }
                frame 57 {
                  n3100 = local write "S 58"(w4138) -> ()
                }
                frame 58 {
                  n3101 = local write "S 59"(w4139) -> ()
                }
                frame 59 {
                  n3102 = local write "S 60"(w4140) -> ()
                }
                frame 60 {
                  n3103 = local write "S 62"(w4141) -> ()
                }
                frame 61 {
                  n3104 = local write "S 63"(w4142) -> ()
                }
                frame 62 {
                  n3105 = local write "S 64"(w4143) -> ()
                }
                frame 63 {
                  n3106 = local write "S 65"(w4144) -> ()
                }
                frame 64 {
                  n3107 = local write "S 66"(w4145) -> ()
                }
                frame 65 {
                  n3108 = local write "S 67"(w4146) -> ()
                }
                frame 66 {
                  n3109 = local write "S 68"(w4147) -> ()
                }
                frame 67 {
                  n3110 = local write "S 69"(w4148) -> ()
                }
                frame 68 {
                  n3111 = local write "S 70"(w4149) -> ()
                }
                frame 69 {
                  n3112 = local write "S 71"(w4150) -> ()
                }
                frame 70 {
                  n3113 = local write "S 72"(w4151) -> ()
                }
                frame 71 {
                  n3114 = local write "S 73"(w4152) -> ()
                }
                frame 72 {
                  n3115 = local write "S 74"(w4153) -> ()
                }
                frame 73 {
                  n3116 = local write "S 75"(w4154) -> ()
                }
                frame 74 {
                  n3117 = local write "S 76"(w4155) -> ()
                }
                frame 75 {
                  n3118 = local write "S 77"(w4156) -> ()
                }
                frame 76 {
                  n3119 = local write "S 78"(w4157) -> ()
                }
                frame 77 {
                  n3120 = local write "S 79"(w4158) -> ()
                }
                frame 79 {
                  n3121 = property on="Sample Temperature ( °C )" class="XYGraph (strict)"("Y Scale.Name Label.Text"=w4159) -> ()  [unwired: 2 in, 2 out]
                }
                frame 80 {
                  n3122 = local write "S 81"(w4160) -> ()
                  n3123 = property on="Humidity ( %RH )" class="XYGraph (strict)"("Y Scale.Name Label.Text"=w4160) -> ()  [unwired: 2 in, 2 out]
                }
                frame 78 {
                  n3124 = property on="Air Temperature  ( °C )" class="XYGraph (strict)"("X Scale.Name Label.Text"=w4161) -> ()  [unwired: 2 in, 2 out]
                  n3125 = property on="Humidity ( %RH )" class="XYGraph (strict)"("X Scale.Name Label.Text"=w4161) -> ()  [unwired: 2 in, 2 out]
                  n3126 = property on="Sample Temperature ( °C )" class="XYGraph (strict)"("X Scale.Name Label.Text"=w4161) -> ()  [unwired: 2 in, 2 out]
                  n3127 = property on="Coefficient Of Friction" class="XYGraph (strict)"("X Scale.Name Label.Text"=w4161) -> ()  [unwired: 2 in, 2 out]
                }
                frame 81 {
